vi "题目3.vi"() -> ()   [LabVIEW 2017]
panel:
  out "添加的数组":dbl[][][](array[numeric])
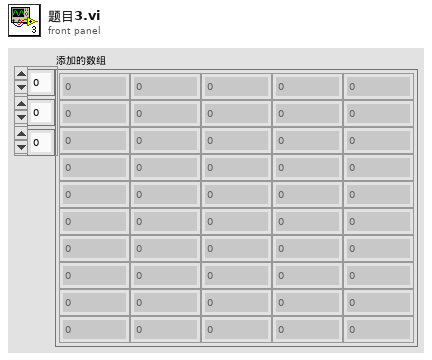
[diagram p1: front panel]
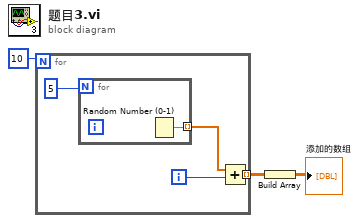
[diagram p0: block diagram]
diagram:
  n1 = for {
    N: 10 -> [_]
    tunnel: [w4] -> w1 mode=indexing
    i -> [w5]
    n2 = for {
      N: 5 -> [_]
      tunnel: [w8] -> w6 mode=indexing
      n3 = Random Number (0-1)() -> (number: 0 to 1=w8:dbl)
    }
    n4 = Add(x=w6, y=w5) -> (x+y=w4:dbl[])
  }
  n5 = Build Array(w1) -> (→"添加的数组":dbl[][][])
